vi "CDL0100 Recipe Creator v1.1.vi"(0 "Previous Recipe Path":path=path "C:/ProgramData/TDK/CDL0100/Recipe.ini") -> (1 "New Recipe Path":path=path "C:/ProgramData/TDK/CDL0100/Recipe.ini", 2 "Rectifier Info Out":dbl[][](array[numeric]), 3 "canceled?":bool)   [LabVIEW 2019]
uses:
  <vilib>/Utility/config.llb/Write Key (String).vi
  <vilib>/Utility/config.llb/Write Key (Double).vi
  <vilib>/Utility/config.llb/Write Key (U32).vi
  <vilib>/Utility/config.llb/Read Key (String).vi
  <vilib>/Utility/config.llb/Read Key (Double).vi
  <vilib>/Utility/config.llb/Read Key (I32).vi
  <vilib>/Utility/config.llb/NI_LVConfig.lvlib
panel:
  in  "Notes":string
  out "Under100":string="! Sum < 100 !"
  out "Over100":string="! Sum > 100 !"
  in  "Constants":cluster{"F":dbl, "n":dbl, "r":dbl, "MW":dbl}={"F"=96485.0, "n"=2.0, "r"=8.95, "MW"=63.546}
  out "Total Amp Min":cluster{"Left (back)":dbl, "Right (front)":dbl}={"Left (back)"=1.15, "Right (front)"=1.15}
  in  "Frame Surface Area (dm^2)":cluster{"Left (back)":dbl, "Right (front)":dbl}={"Left (back)"=1.15, "Right (front)"=1.15}
  out "Plating Time":string
  out "Recipe Time\n(min)":dbl[][](array[numeric]) format="%#_4g"
  out "Rectifier Setpoints":dbl[][](array[numeric]) format="%.1f"
  in  "Plating Thickness (um)":cluster{"Left (back)":dbl, "Right (front)":dbl}
  in  "Surface Area (mm^2)":cluster{"Left (back)":dbl, "Right (front)":dbl}
  in  "Plating Steps":u32=1 min=1 max=5 step=1
  in  "New Version":i32
  in  "New Recipe Name":string
  in  "Recipe":dbl[][](array[numeric])
  in  "cancel":bool
  out "Previous Version":i32
  out "Previous Recipe Name":string
  in  "Save":bool
  # "LEFT (back)"
  # "RIGHT (front)"
  # "% of Plating"
  # "ASD"
  # "Amps"
  # "AmpMin"
  # "Amps"
  # "AmpMin"
  # "Left"
  # "Right"
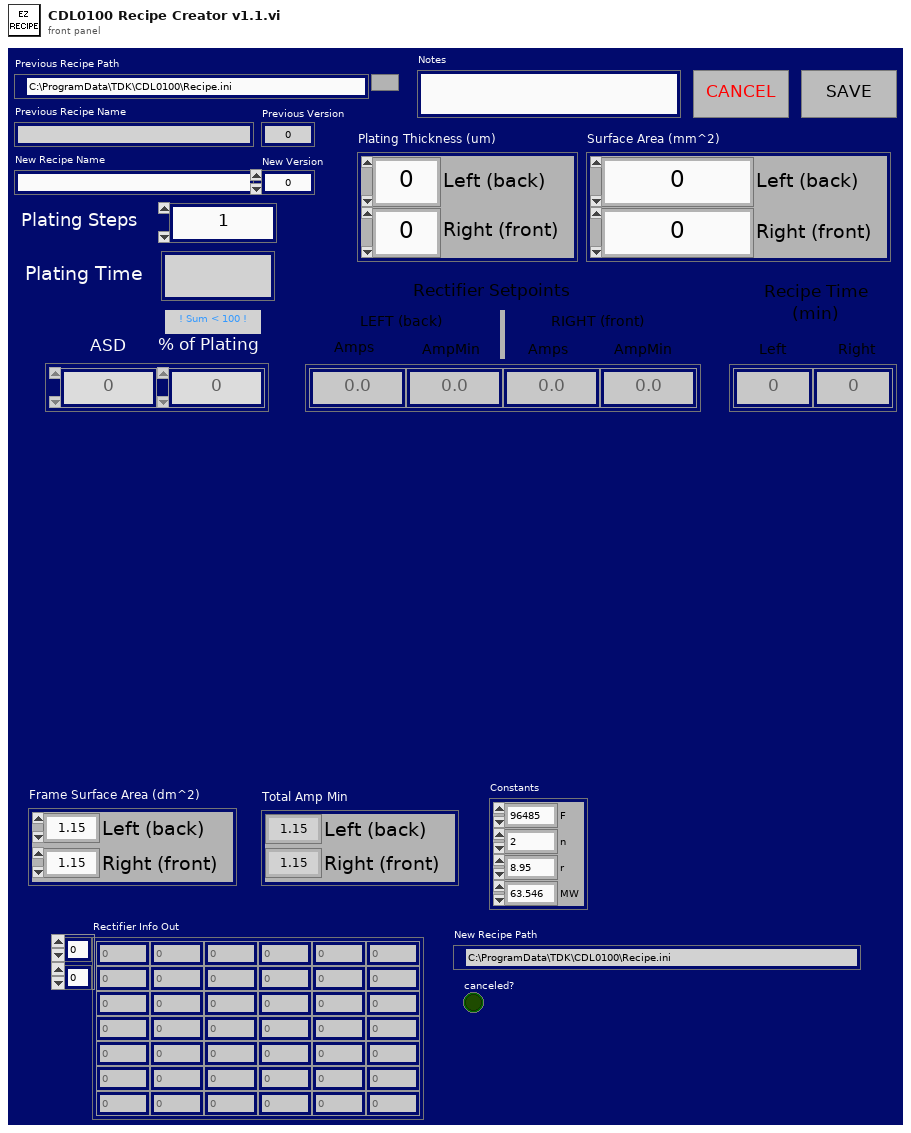
[diagram p1: front panel]
types:
  T1 = typedef "NI_LVConfig.lvlib/Config Data RefNum.ctl" = refnum<k1>
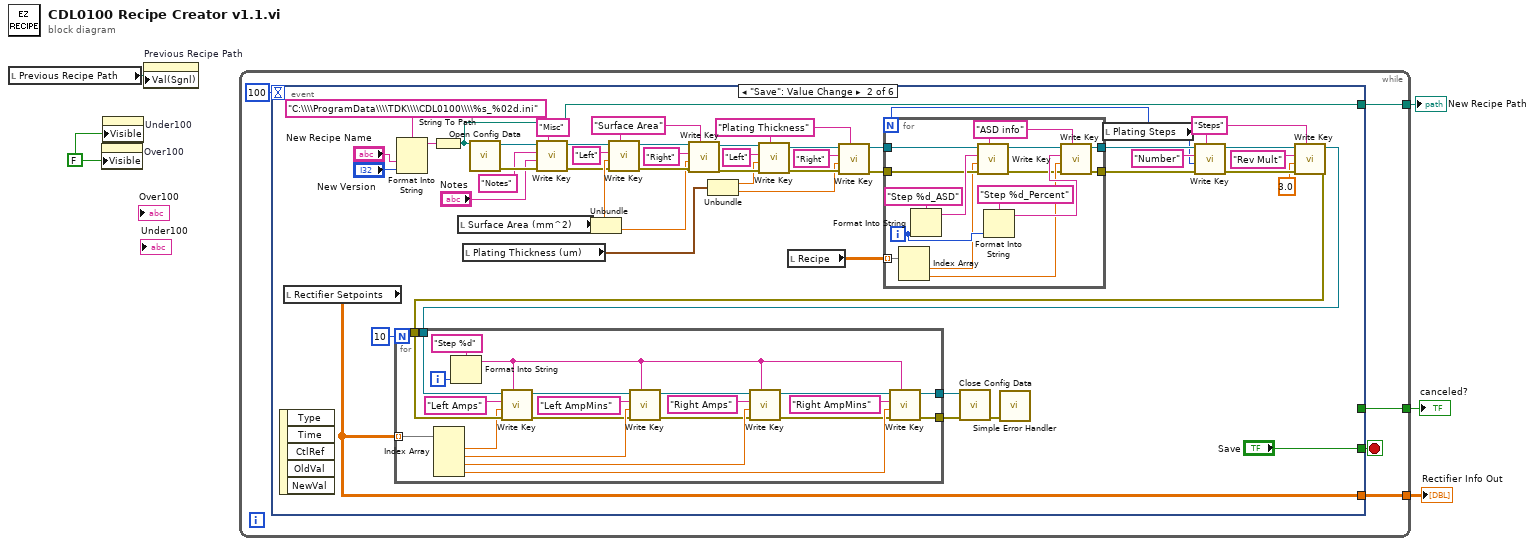
[diagram p0: block diagram]
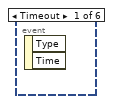
[diagram p2: hidden frame]
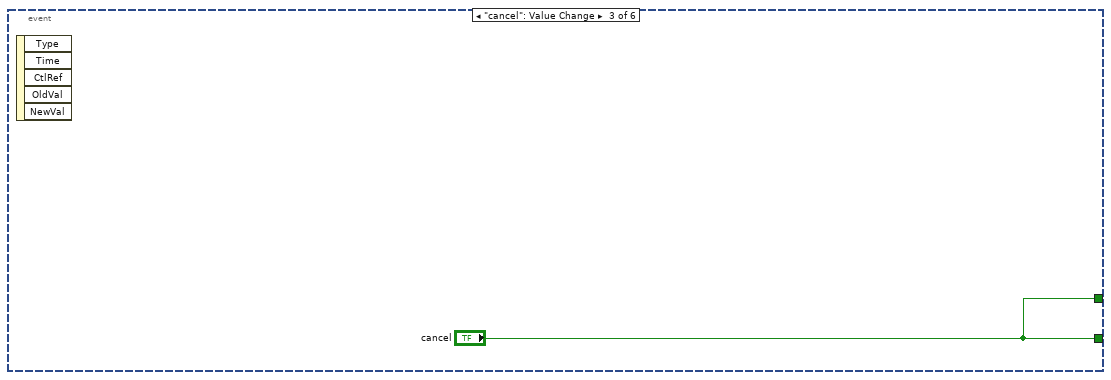
[diagram p3: hidden frame]
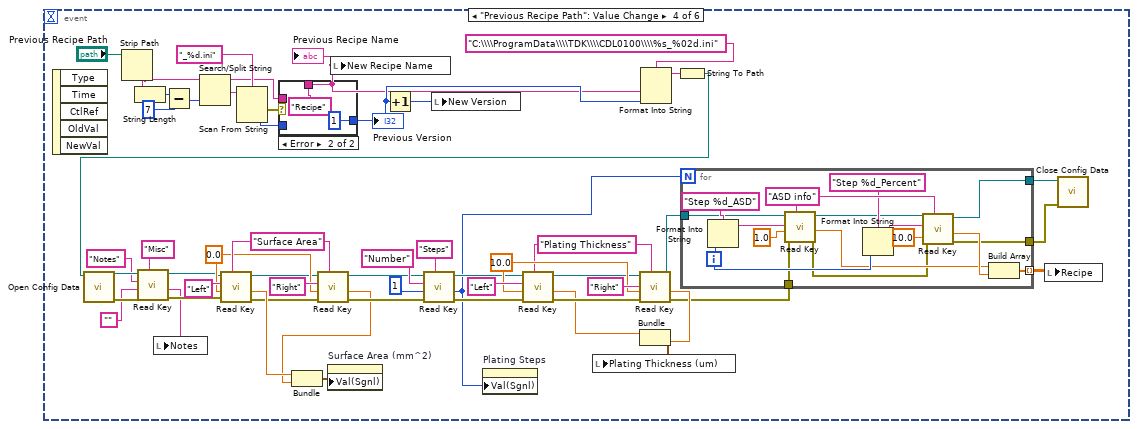
[diagram p4: hidden frame]
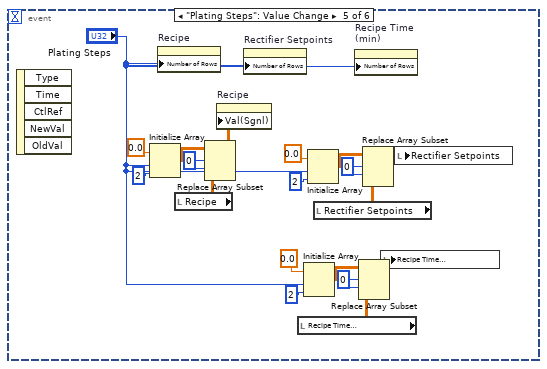
[diagram p6: hidden frame]
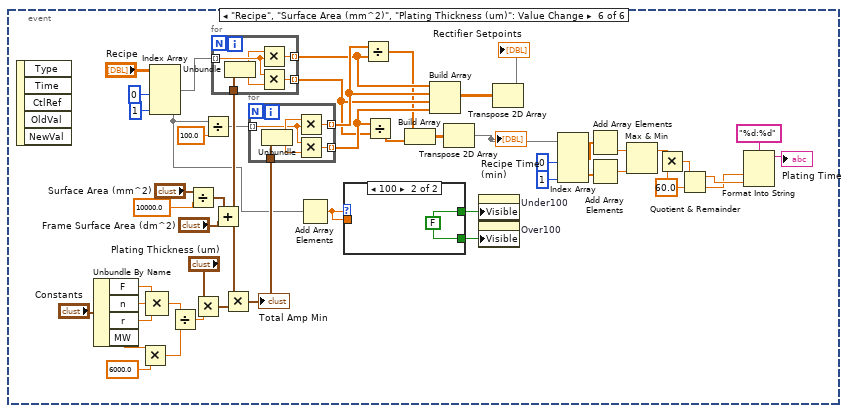
[diagram p7: hidden frame]
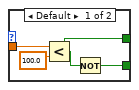
[diagram p8: hidden frame]
diagram:
  w1 = FALSE ("Visible")
  n1 = local read "Previous Recipe Path"() -> (w5:path)
  n2 = property on="Over100" class="Str"("Visible"=w1) -> ()  [unwired: 2 in, 2 out]
  n3 = property on="Under100" class="Str"("Visible"=w1) -> ()  [unwired: 2 in, 2 out]
  n4 = property on="Previous Recipe Path" class="Path"("Val(Sgnl)"=w5) -> ()  [unwired: 2 in, 2 out]
  n5 = while {
    tunnel: [w8] -> w4
    tunnel: [w7] -> w3
    tunnel: [w6] -> w2
    stop <- w10 stop-if-true
    n6 = event shown="[1] \"Save\": Value Change" {
      selector: _ -> [_ _ _ _ _ _]
      dyn-events: _ -> [_ _ _ _ _ _]
      timeout: 100 -> [_ _ _ _ _ _]
      tunnel: [_ "Save" "cancel" _ _ _] -> w10
      tunnel: [_ w23 _ _ _ _] -> w8
      tunnel: [_ _ "cancel" _ _ _] -> w7
      tunnel: [_ w18 _ _ _ _] -> w6
      event Timeout {
        n7 = event-data() -> ()  [unwired: 1 in, 2 out]
      }
      event "Save": Value Change {
        w44 = "Plating Thickness" ("section")
        w24 = "Steps" ("section")
        w57 = "Surface Area" ("section")
        n8 = event-data() -> ()  [unwired: 1 in, 5 out]
        n9 = local read "Rectifier Setpoints"() -> (w23:dbl[][])
        n10 = Format Into String(format string="C:\\\\ProgramData\\\\TDK\\\\CDL0100\\\\%s_%02d.ini", "New Recipe Name", "New Version") -> (resulting string=w58:string)  [unwired: 2 in, 1 out]
        n11 = String To Path(string=w58) -> (path=w18:path)
        n12 = local read "Surface Area (mm^2)"() -> (w53:cluster{"Left (back)":dbl, "Right (front)":dbl})
        n13 = local read "Plating Thickness (um)"() -> (w37:cluster{"Left (back)":dbl, "Right (front)":dbl})
        n14 = call <vilib>:"Open Config Data.vi"("configuration file path"=w18) -> ("error out"=w15:errorcluster, "refnum"=w17:T1)  [unwired: 8 in, 1 out]
        n15 = call-poly <vilib>:"Write Key.vi"("section"="Misc", "error in (no error)"=w15, "value"="Notes", "key"="Notes" ("section"), "refnum"=w17) -> ("error out"=w14:errorcluster, "refnum out"=w16:T1)  [unwired: 4 in, 1 out]
        n16 = Unbundle(w53) -> ("Left (back)"=w52:dbl, "Right (front)"=w51:dbl)
        n17 = call-poly <vilib>:"Write Key.vi"("section"=w57, "error in (no error)"=w14, "value"=w52, "key"="Left" ("section"), "refnum"=w16) -> ("error out"=w54:errorcluster, "refnum out"=w55:T1)  [unwired: 4 in, 1 out]
        n18 = call-poly <vilib>:"Write Key.vi"("section"=w57, "error in (no error)"=w54, "value"=w51, "key"="Right" ("section"), "refnum"=w55) -> ("error out"=w40:errorcluster, "refnum out"=w39:T1)  [unwired: 4 in, 1 out]
        n19 = Unbundle(w37) -> ("Left (back)"=w36:dbl, "Right (front)"=w35:dbl)
        n20 = call-poly <vilib>:"Write Key.vi"("section"=w44, "error in (no error)"=w40, "value"=w36, "key"="Left" ("section"), "refnum"=w39) -> ("error out"=w41:errorcluster, "refnum out"=w42:T1)  [unwired: 4 in, 1 out]
        n21 = local read "Recipe"() -> (w22:dbl[][])
        n22 = call-poly <vilib>:"Write Key.vi"("section"=w44, "error in (no error)"=w41, "value"=w35, "key"="Right" ("section"), "refnum"=w42) -> ("error out"=w33:errorcluster, "refnum out"=w34:T1)  [unwired: 4 in, 1 out]
        n23 = local read "Plating Steps"() -> (w30:u32)
        n24 = for {
          N: w30 -> [_]
          tunnel: w34 -> [w96]
          tunnel: w33 -> [w94]
          tunnel: w22 -> [w90] mode=indexing
          tunnel: [w84] -> w31
          tunnel: [w83] -> w32
          i -> [w93]
          w85 = "ASD info" ("format string")
          n25 = Index Array(array=w90) -> (element #1=w89:dbl, element #2=w88:dbl)  [unwired: 2 in]
          n26 = Format Into String(format string="Step %d_ASD", w93) -> (resulting string=w95:string)  [unwired: 2 in, 1 out]
          n27 = call-poly <vilib>:"Write Key.vi"("section"=w85, "error in (no error)"=w94, "value"=w89, "key"=w95, "refnum"=w96) -> ("error out"=w87:errorcluster, "refnum out"=w86:T1)  [unwired: 4 in, 1 out]
          n28 = Format Into String(format string="Step %d_Percent", w93) -> (resulting string=w91:string)  [unwired: 2 in, 1 out]
          n29 = call-poly <vilib>:"Write Key.vi"("section"=w85, "error in (no error)"=w87, "value"=w88, "key"=w91, "refnum"=w86) -> ("error out"=w84:errorcluster, "refnum out"=w83:T1)  [unwired: 4 in, 1 out]
        }
        n30 = call-poly <vilib>:"Write Key.vi"("section"=w24, "error in (no error)"=w31, "value"=w30, "key"="Number" ("section"), "refnum"=w32) -> ("error out"=w48:errorcluster, "refnum out"=w47:T1)  [unwired: 4 in, 1 out]
        n31 = call-poly <vilib>:"Write Key.vi"("section"=w24, "error in (no error)"=w48, "value"=3.0 ("Right (front)"), "key"="Rev Mult" ("section"), "refnum"=w47) -> ("error out"=w27:errorcluster, "refnum out"=w28:T1)  [unwired: 4 in, 1 out]
        n32 = for {
          N: 10 -> [_]
          tunnel: w23 -> [w82] mode=indexing
          tunnel: w28 -> [w81]
          tunnel: w27 -> [w80]
          tunnel: [w62] -> w26
          tunnel: [w61] -> w25
          i -> [w78]
          n33 = Index Array(array=w82) -> (element #1=w73:dbl, element #2=w68:dbl, element #3=w67:dbl, element #4=w66:dbl)  [unwired: 4 in]
          n34 = Format Into String(format string="Step %d", w78) -> (resulting string=w71:string)  [unwired: 2 in, 1 out]
          n35 = call-poly <vilib>:"Write Key.vi"("section"=w71, "error in (no error)"=w80, "value"=w73, "key"="Left Amps" ("format string"), "refnum"=w81) -> ("error out"=w63:errorcluster, "refnum out"=w76:T1)  [unwired: 4 in, 1 out]
          n36 = call-poly <vilib>:"Write Key.vi"("section"=w71, "error in (no error)"=w63, "value"=w68, "key"="Left AmpMins" ("format string"), "refnum"=w76) -> ("error out"=w64:errorcluster, "refnum out"=w75:T1)  [unwired: 4 in, 1 out]
          n37 = call-poly <vilib>:"Write Key.vi"("section"=w71, "error in (no error)"=w64, "value"=w67, "key"="Right Amps" ("format string"), "refnum"=w75) -> ("error out"=w65:errorcluster, "refnum out"=w74:T1)  [unwired: 4 in, 1 out]
          n38 = call-poly <vilib>:"Write Key.vi"("section"=w71, "error in (no error)"=w65, "value"=w66, "key"="Right AmpMins" ("format string"), "refnum"=w74) -> ("error out"=w62:errorcluster, "refnum out"=w61:T1)  [unwired: 4 in, 1 out]
        }
        n39 = call <vilib>:"Close Config Data.vi"("error in (no error)"=w26, "refnum"=w25) -> ("error out"=w21:errorcluster)  [unwired: 8 in, 1 out]
        n40 = call <vilib>:"Simple Error Handler.vi"("error in (no error)"=w21) -> ()  [unwired: 4 in, 5 out]
      }
      event "cancel": Value Change {
        n41 = event-data() -> ()  [unwired: 1 in, 5 out]
      }
      event "Previous Recipe Path": Value Change {
        w131 = 10.0 ("default value")
        w124 = 0.0 ("default value")
        w130 = "Plating Thickness" ("section")
        w125 = "Surface Area" ("section")
        n42 = event-data() -> ()  [unwired: 1 in, 5 out]
        n43 = Strip Path(path="Previous Recipe Path") -> (name=w153:string)  [unwired: 1 out]
        n44 = String Length(string=w153) -> (length=w152:i32)
        n45 = Subtract(x=w152, y=7) -> (x-y=w148:i32)
        n46 = Search/Split String(string=w153, offset (0)=w148) -> (substring before match=w146:string, match + rest of string=w150:string)  [unwired: 1 in, 1 out]
        n47 = Scan From String(format string="_%d.ini", input string=w150) -> (error out=w145:errorcluster, output 1=w147:i32)  [unwired: 3 in, 2 out]
        n48 = case shown="Error" w145 {
          tunnel: w147 -> [w171 _]
          tunnel: w146 -> [w172 _]
          tunnel: [w172 "Recipe" ("name")] -> w110
          tunnel: [w171 1] -> w111
          frame No Error {
          }
          frame Error {
          }
        }
        "Previous Recipe Name" <- w110
        "Previous Version" <- w111
        n49 = local write "New Recipe Name"(w110) -> ()
        n50 = Increment(x=w111) -> (x+1=w112:i32)
        n51 = local write "New Version"(w112) -> ()
        n52 = Format Into String(format string="C:\\\\ProgramData\\\\TDK\\\\CDL0100\\\\%s_%02d.ini", w110, w111) -> (resulting string=w113:string)  [unwired: 2 in, 1 out]
        n53 = String To Path(string=w113) -> (path=w107:path)
        n54 = call <vilib>:"Open Config Data.vi"("configuration file path"=w107) -> ("error out"=w103:errorcluster, "refnum"=w105:T1)  [unwired: 8 in, 1 out]
        n55 = call-poly <vilib>:"Read Key.vi"("section"="Misc", "error in (no error)"=w103, "default value"="", "key"="Notes", "refnum"=w105) -> ("error out"=w102:errorcluster, "value"=w99:string, "refnum out"=w104:T1)  [unwired: 3 in, 1 out]
        n56 = local write "Notes"(w99) -> ()
        n57 = call-poly <vilib>:"Read Key.vi"("section"=w125, "error in (no error)"=w102, "default value"=w124, "key"="Left", "refnum"=w104) -> ("error out"=w122:errorcluster, "value"=w142:dbl, "refnum out"=w123:T1)  [unwired: 3 in, 1 out]
        n58 = call-poly <vilib>:"Read Key.vi"("section"=w125, "error in (no error)"=w122, "default value"=w124, "key"="Right", "refnum"=w123) -> ("error out"=w121:errorcluster, "value"=w118:dbl, "refnum out"=w120:T1)  [unwired: 3 in, 1 out]
        n59 = Bundle("value"=w142, "value"=w118) -> (w141:cluster{"value":dbl, "value":dbl})  [unwired: 1 in]
        n60 = property on="Surface Area (mm^2)" class="Clust (strict)"("Val(Sgnl)"=w141) -> ()  [unwired: 2 in, 2 out]
        n61 = call-poly <vilib>:"Read Key.vi"("section"="Steps", "error in (no error)"=w121, "default value"=1 ("value"), "key"="Number", "refnum"=w120) -> ("error out"=w133:errorcluster, "value"=w117:i32, "refnum out"=w126:T1)  [unwired: 3 in, 1 out]
        n62 = property on="Plating Steps" class="DigNum (strict)"("Val(Sgnl)"=w117) -> ()  [unwired: 2 in, 2 out]
        n63 = call-poly <vilib>:"Read Key.vi"("section"=w130, "error in (no error)"=w133, "default value"=w131, "key"="Left", "refnum"=w126) -> ("error out"=w132:errorcluster, "value"=w128:dbl, "refnum out"=w129:T1)  [unwired: 3 in, 1 out]
        n64 = call-poly <vilib>:"Read Key.vi"("section"=w130, "error in (no error)"=w132, "default value"=w131, "key"="Right", "refnum"=w129) -> ("error out"=w115:errorcluster, "value"=w127:dbl, "refnum out"=w116:T1)  [unwired: 3 in, 1 out]
        n65 = Bundle("value"=w128, "value"=w127) -> (w135:cluster{"value":dbl, "value":dbl})  [unwired: 1 in]
        n66 = local write "Plating Thickness (um)"(w135) -> ()
        n67 = for {
          N: w117 -> [_]
          tunnel: [w160] -> w114 mode=indexing
          tunnel: [w158] -> w134
          tunnel: [w157] -> w119
          tunnel: w116 -> [w156]
          tunnel: w115 -> [w154]
          i -> [w166]
          w167 = "ASD info" ("section")
          n68 = Format Into String(format string="Step %d_ASD", w166) -> (resulting string=w169:string)  [unwired: 2 in, 1 out]
          n69 = call-poly <vilib>:"Read Key.vi"("section"=w167, "error in (no error)"=w154, "default value"=1.0, "key"=w169, "refnum"=w156) -> ("error out"=w159:errorcluster, "value"=w161:dbl, "refnum out"=w155:T1)  [unwired: 3 in, 1 out]
          n70 = Format Into String(format string="Step %d_Percent", w166) -> (resulting string=w164:string)  [unwired: 2 in, 1 out]
          n71 = call-poly <vilib>:"Read Key.vi"("section"=w167, "error in (no error)"=w159, "default value"=10.0, "key"=w164, "refnum"=w155) -> ("error out"=w158:errorcluster, "value"=w162:dbl, "refnum out"=w157:T1)  [unwired: 3 in, 1 out]
          n72 = Build Array(w161, w162) -> (w160:dbl[])
        }
        n73 = local write "Recipe"(w114) -> ()
        n74 = call <vilib>:"Close Config Data.vi"("error in (no error)"=w134, "refnum"=w119) -> ()  [unwired: 8 in, 2 out]
      }
      event "Plating Steps": Value Change {
        w181 = 0 ("index (row)")
        w188 = 0 ("index (row)")
        w190 = 0 ("index (row)")
        n75 = event-data() -> ()  [unwired: 1 in, 5 out]
        n76 = Initialize Array(0.0, "Plating Steps", 2 ("dimension size")) -> (w191:dbl[][])
        n77 = property on="Recipe" class="Arr (strict)"("Number of Rows"="Plating Steps") -> ()  [unwired: 2 in, 2 out]
        n78 = local read "Recipe"() -> (w189:dbl[][])
        n79 = Replace Array Subset(array=w191, new element=w189, index (row)=w190, index (col)=w190) -> (w175:dbl[][])
        n80 = property on="Recipe" class="Arr (strict)"("Val(Sgnl)"=w175) -> ()  [unwired: 2 in, 2 out]
        n81 = property on="Rectifier Setpoints" class="Arr (strict)"("Number of Rows"="Plating Steps") -> ()  [unwired: 2 in, 2 out]
        n82 = local read "Recipe Time\n(min)"() -> (w180:dbl[][])
        n83 = Initialize Array(0.0, "Plating Steps", 2 ("dimension size")) -> (w182:dbl[][])
        n84 = Initialize Array(0.0, "Plating Steps", 2 ("dimension size")) -> (w187:dbl[][])
        n85 = local read "Rectifier Setpoints"() -> (w177:dbl[][])
        n86 = property on="Recipe Time\n(min)" class="Arr (strict)"("Number of Rows"="Plating Steps") -> ()  [unwired: 2 in, 2 out]
        n87 = Replace Array Subset(array=w182, new element=w180, index (row)=w181, index (col)=w181) -> (w179:dbl[][])
        n88 = Replace Array Subset(array=w187, new element=w177, index (row)=w188, index (col)=w188) -> (w176:dbl[][])
        n89 = local write "Recipe Time\n(min)"(w179) -> ()
        n90 = local write "Rectifier Setpoints"(w176) -> ()
      }
      event "Recipe", "Surface Area (mm^2)", "Plating Thickness (um)": Value Change {
        w200 = 60.0 ("y")
        n91 = event-data() -> ()  [unwired: 1 in, 5 out]
        n92 = Unbundle By Name("Constants") -> ("F"=w238:dbl, "n"=w237:dbl, "r"=w236:dbl, "MW"=w235:dbl)
        n93 = Multiply(x=w235, y=6000.0) -> (x*y=w232:dbl)
        n94 = Compound Arithmetic op=MULTIPLY(w238, w237, w236) -> (w233:dbl)
        n95 = Index Array(array="Recipe", index (col) #1=0 ("disabled index (col)"), index (col) #2=1 ("index (col)")) -> (element #1=w227:dbl[], element #2=w195:dbl[])  [unwired: 2 in]
        n96 = Divide(x=w233, y=w232) -> (x/y=w230:dbl)
        n97 = Divide(x="Surface Area (mm^2)", y=10000.0) -> (x/y=w240:cluster{"Left (back)":dbl, "Right (front)":dbl})
        n98 = Multiply(x="Plating Thickness (um)", y=w230) -> (x*y=w229:cluster{"Left (back)":dbl, "Right (front)":dbl})
        n99 = Divide(x=w195, y=100.0) -> (x/y=w194:dbl[])
        n100 = Add(x=w240, y="Frame Surface Area (dm^2)") -> (x+y=w226:cluster{"Left (back)":dbl, "Right (front)":dbl})
        n101 = for {
          tunnel: w227 -> [w259] mode=indexing
          tunnel: w226 -> [w260]
          tunnel: [w256] -> w218 mode=indexing
          tunnel: [w255] -> w216 mode=indexing
          n102 = Unbundle(w260) -> ("Left (back)"=w257:dbl, "Right (front)"=w258:dbl)
          n103 = Multiply(x=w257, y=w259) -> (x*y=w256:dbl)
          n104 = Multiply(x=w259, y=w258) -> (x*y=w255:dbl)
        }
        n105 = Multiply(x=w226, y=w229) -> (x*y=w224:cluster{"Left (back)":dbl, "Right (front)":dbl})
        "Total Amp Min" <- w224
        n106 = for {
          tunnel: w194 -> [w249] mode=indexing
          tunnel: w224 -> [w254]
          tunnel: [w251] -> w219 mode=indexing
          tunnel: [w250] -> w217 mode=indexing
          n107 = Unbundle(w254) -> ("Left (back)"=w252:dbl, "Right (front)"=w253:dbl)
          n108 = Multiply(x=w252, y=w249) -> (x*y=w251:dbl)
          n109 = Multiply(x=w249, y=w253) -> (x*y=w250:dbl)
        }
        n110 = Add Array Elements(numeric array=w195) -> (sum=w198:dbl)
        n111 = case shown="100" w198 {
          tunnel: w198 -> [w247 _]
          tunnel: [w245 w248] -> w197
          tunnel: [w244 w248] -> w196
          frame Default {
            n112 = Less?(x=w247, y=100.0) -> (x < y?=w245:bool)
            n113 = Not(x=w245) -> (.not. x?=w244:bool)
          }
          frame 100 {
            w248 = FALSE ("Visible")
          }
        }
        n114 = Divide(x=w219, y=w218) -> (x/y=w215:dbl[])
        n115 = Divide(x=w217, y=w216) -> (x/y=w214:dbl[])
        n116 = Build Array(w215, w214) -> (w213:dbl[][])
        n117 = Build Array(w218, w219, w216, w217) -> (w221:dbl[][])
        n118 = Transpose 2D Array(2D array=w213) -> (transposed array=w212:dbl[][])
        "Recipe Time\n(min)" <- w212
        n119 = property on="Under100" class="Str"("Visible"=w197) -> ()  [unwired: 2 in, 2 out]
        n120 = property on="Over100" class="Str"("Visible"=w196) -> ()  [unwired: 2 in, 2 out]
        n121 = Transpose 2D Array(2D array=w221) -> (transposed array=→"Rectifier Setpoints":dbl[][])
        n122 = Index Array(array=w212, index (col) #1=0 ("disabled index (col)"), index (col) #2=1 ("index (col)")) -> (element #1=w208:dbl[], element #2=w209:dbl[])  [unwired: 2 in]
        n123 = Add Array Elements(numeric array=w208) -> (sum=w207:dbl)
        n124 = Add Array Elements(numeric array=w209) -> (sum=w206:dbl)
        n125 = Max & Min(x=w207, y=w206) -> (max(x,y)=w202:dbl)  [unwired: 1 out]
        n126 = Multiply(x=w202, y=w200) -> (x*y=w201:dbl)
        n127 = Quotient & Remainder(x=w201, y=w200) -> (x-y*floor(x/y)=w205:dbl, floor(x/y)=w199:dbl)
        n128 = Format Into String(format string="%d:%d" ("time format string (%c)"), w199, w205) -> (resulting string=→"Plating Time":string)  [unwired: 2 in, 1 out]
      }
    }
  }
  "Rectifier Info Out" <- w4
  "canceled?" <- w3
  "New Recipe Path" <- w2
